vi "SLL DE Start AO Task.vi"(8 "error in (no error)":errorcluster, 11 "Array of AO Task":refnum<k21>[](array[refnum])) -> (0 "error out":errorcluster, 3 "Array of AO Task Out":refnum<k21>[](array[refnum]))   [LabVIEW 2013]
doc: "Copyright © 2005, Soliton Technologies.\nAll rights reserved."
uses:
  Controls/SLL DE DAQ Parameters LV2Global Options.ctl
  <vilib>/DAQmx/configure/timing.llb/DAQmx Timing (Sample Clock).vi
  <resource>/objmgr/daqmx.rc
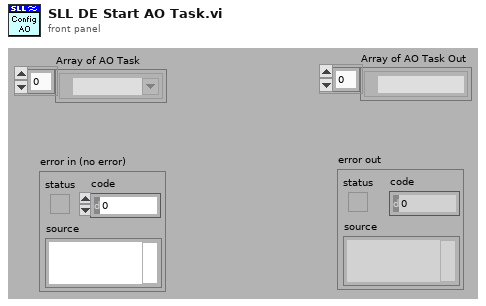
[diagram p1: front panel]
types:
  T1 = typedef "SLL DE DAQ Parameters LV2Global Options.ctl" = enum16{"Read", "Write"}
  T2 = typedef "SLL DE DAQ Engine Parameters.ctl" = cluster{"Enable Engines":cluster{"AI Enable":bool, "AO Enable":bool, "DI Enable":bool, "DO Enable":bool}, "DAQ Control Type":cluster{"Analog Input":enum16{"Finite", "Continuous", "Driver"}, "Analog Output":enum16{"Finite", "Continuous", "Driver"}, "Digital Input":enum16{"Finite", "Continuous", "Driver"}, "Digital Output":enum16{"Finite", "Continuous", "Driver"}}, "DAQ Parameters":cluster{"AI Sampling Rate (Samples/Sec)":dbl, "MvgAVG Window Size (# of Points)":i32, "Enable Filter":bool, "Enable MvgAVG":bool, "Circular Buffer Size (Sec)":dbl, "AO Sampling Rate (Samples/Sec)":dbl, "Graph Update Rate (Samples/Sec)":dbl, "File Logging Rate (Samples/Sec)":i32}, "AO Safe Values":cluster{"Analog Outputs Name":T3, "Analog Outputs Safe Value":dbl}[], "DO Safe Values":cluster{"Digital Outputs Name":T4, "Digital Outputs Safe Value":bool}[], "DO Interconnected Lines":cluster{"First DO Line":string, "Second DO Line":string}[], "AI Channels Unit":cluster{"Channel Name":T5, "Channel Type":T6}[], "Units Information":cluster{"Channel Type":T6, "Unit Text":string, "Maximum":dbl, "Minmum":dbl, "Increments":dbl}[]}
  T3 = typedef "SLL DE List of Analog Outputs.ctl" = enum16{"None"}
  T4 = typedef "SLL DE List of Digital Outputs.ctl" = enum16{"STATION1_START TEST", "STATION1_STOP TEST", "STATION1_LIGHT1", "STATION1_LIGHT2", "STATION1_LIGHT3", "STATION1_SELECT_TEST", "STATION2_START TEST", "STATION2_STOP TEST", "STATION2_LIGHT1", "STATION2_LIGHT2", "STATION2_LIGHT3", "STATION2_SELECT_TEST", "STATION3_START TEST", "STATION3_STOP TEST", "STATION3_LIGHT1", "STATION3_LIGHT2", "STATION3_LIGHT3", "STATION3_SELECT_TEST", "STATION4_START TEST", "STATION4_STOP TEST", "STATION4_LIGHT1", "STATION4_LIGHT2", "STATION4_LIGHT3", "STATION4_SELECT_TEST"}
  T5 = typedef "SLL DE List of Analog Inputs.ctl" = enum16{"None"}
  T6 = typedef "SLL DE List of AI Channel Type.ctl" = enum16{"Pressure", "Flow", "Temperature", "Time Scale", "Voltage", "Current", "Frequency", "Sound", "Speed", "Torque", "Distance", "Channel Type 1", "Channel Type 2", "Channel Type 3"}
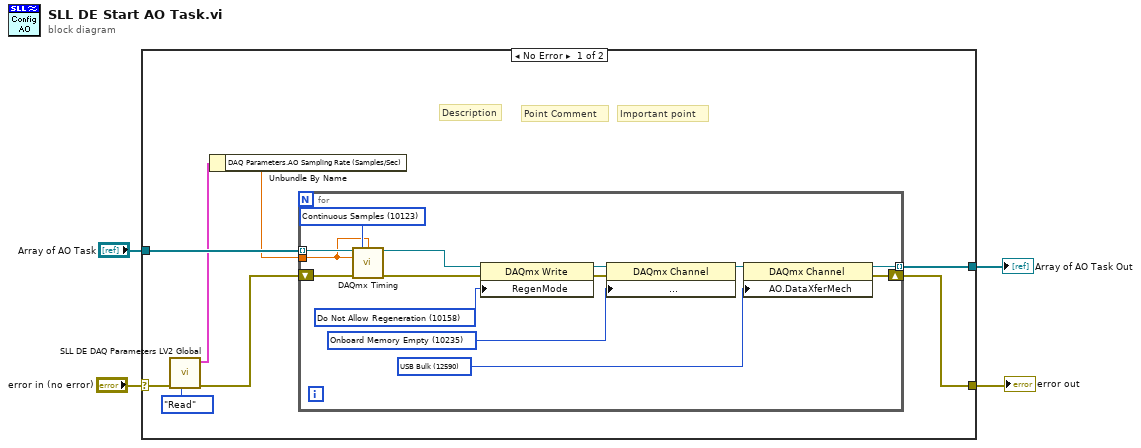
[diagram p0: block diagram]
diagram:
  n1 = case shown="No Error" "error in (no error)" {
    selector: "error in (no error)" -> [w8 w28]
    tunnel: [w6 w28] -> w3
    tunnel: "Array of AO Task" -> [w12 w27]
    tunnel: [w5 w27] -> w1
    frame No Error {
      # "Point Comment"
      # "Important point"
      # "Description"
      n2 = call "SLL DE DAQ Parameters LV2 Global.vi"("Option"=SLL_DE_DAQ_Parameters_LV2Global_Options."Read", "Error in (no error)"=w8) -> ("Error out"=w7:errorcluster, "Global Info"=w10:T2)  [unwired: 8 in]
      n3 = Unbundle By Name(w10) -> ("DAQ Parameters.AO Sampling Rate (Samples/Sec)"=w9:dbl)
      n4 = for {
        tunnel: w9 -> [w23]
        shift-right: [w15] -> w6
        shift-left: w7 -> [w26]
        tunnel: w12 -> [w25] mode=indexing
        tunnel: [w13] -> w5 mode=indexing
        w14 = 12590 items=["DMA"=10054, "Interrupts"=10204, "Programmed I/O"=10264, "USB Bulk"=12590] ("AO.DataXferMech")
        w17 = 10235 items=["Onboard Memory Empty"=10235, "Onboard Memory Half Full or Less"=10239, "Onboard Memory Less than Full"=10242] ("AO.DataXferReqCond")
        w22 = 10158 items=["Allow Regeneration"=10097, "Do Not Allow Regeneration"=10158] ("RegenMode")
        w24 = 10123 items=["Finite Samples"=10178, "Continuous Samples"=10123, "Hardware Timed Single Point"=12522] ("sample mode")
        n5 = call-poly <vilib>:"DAQmx Timing.vi"("task/channels in"=w25, "sample mode"=w24, "samples per channel"=w23, "rate"=w23, "error in"=w26) -> ("task out"=w21:refnum<k21>, "error out"=w20:errorcluster)  [unwired: 2 in, 7 out]
        n6 = property class="DAQmx Write"(reference=w21, error in=w20, "RegenMode"=w22) -> (reference out=w19:refnum<k21>, error out=w18:errorcluster)
        n7 = property class="DAQmx Channel"(reference=w19, error in=w18, "Analog Output:General Properties:Advanced:Data Transfer and Memory:Data Transfer Request Condition"=w17) -> (reference out=w16:refnum<k21>)  [unwired: 1 out]
        n8 = property class="DAQmx Channel"(reference=w16, "AO.DataXferMech"=w14) -> (reference out=w13:refnum<k21>, error out=w15:errorcluster)  [unwired: 1 in]
      }
    }
    frame Error {
    }
  }
  "error out" <- w3
  "Array of AO Task Out" <- w1
